vi "Same name VI.vi"(8 "error in (no error)":errorcluster, 9 "Numeric":dbl=4.0, 11 "BaseClass in":refnum<class "BaseClass.lvclass">) -> (0 "error out":errorcluster, 1 "Numeric 2":dbl, 3 "BaseClass out":refnum<class "BaseClass.lvclass">)   [LabVIEW 2022 SP3, in "BaseClass.lvclass"]
uses:
  BaseClass.lvclass
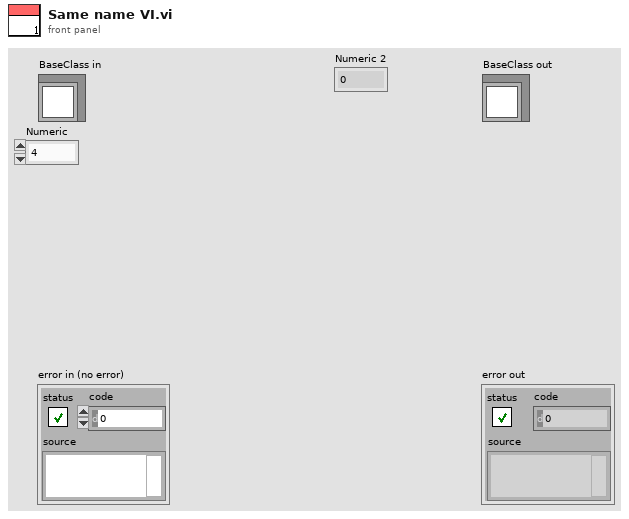
[diagram p1: front panel]
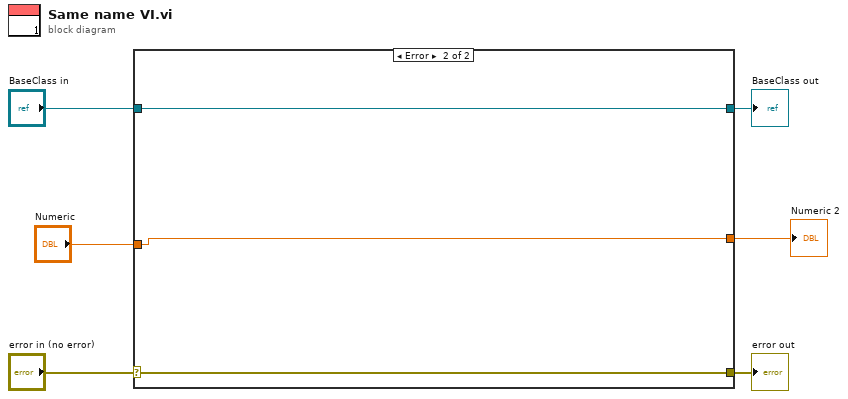
[diagram p0: block diagram]
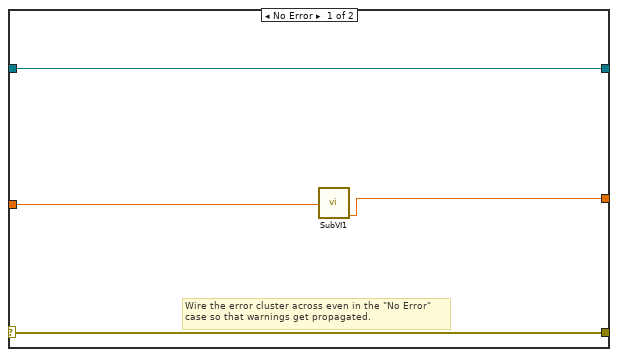
[diagram p2: hidden frame]
diagram:
  n1 = case shown="Error" "error in (no error)" {
    selector: "error in (no error)" -> [w9 w13]
    tunnel: [w9 w13] -> w5
    tunnel: [w10 w12] -> w3
    tunnel: "BaseClass in" -> [w10 w12]
    tunnel: "Numeric" -> [w8 w11]
    tunnel: [w7 w11] -> w1
    frame No Error {
      # "Wire the error cluster across even in the \"No Error\"\ncase so that warnings get propagated."
      n2 = call "SubVI1.vi"("x"=w8) -> ("x+y"=w7:dbl)  [unwired: 10 in]
    }
    frame Error {
    }
  }
  "error out" <- w5
  "BaseClass out" <- w3
  "Numeric 2" <- w1
